vi "white line 2.vi"   [LabVIEW 2010, in "Line Follower.lvrbt"]
uses:
  Line Follower.lvrbt
  <vilib>/NXT/Subs/MotorOutput.ctl
  <vilib>/NXT/Block Support/NXT_InputPort.ctl
  <vilib>/NXT/Dual Mode Library/Sensors/Light_On.vi
  <vilib>/NXT/Dual Mode Library/Display/drawNumber.vi
  <vilib>/NXT/Dual Mode Library/Waits/Wait_Num(msec).vi
  <vilib>/NXT/Dual Mode Library/Motors/MotorOn.vi
  <vilib>/NXT/Dual Mode Library/Motors/MotorBrake.vi
  <vilib>/NXT/Dual Mode Library/Sound/Tone.vi
  <vilib>/NXT/Dual Mode Library/Sensors/Sonar_cm.vi
types:
  T1 = typedef "LVHSConnector.ctl" = cluster{"Hardware":string, "Flattened String":string}
  T2 = typedef "MotorOutput.ctl" = u8
  T3 = typedef "NXT_InputPort.ctl" = u8
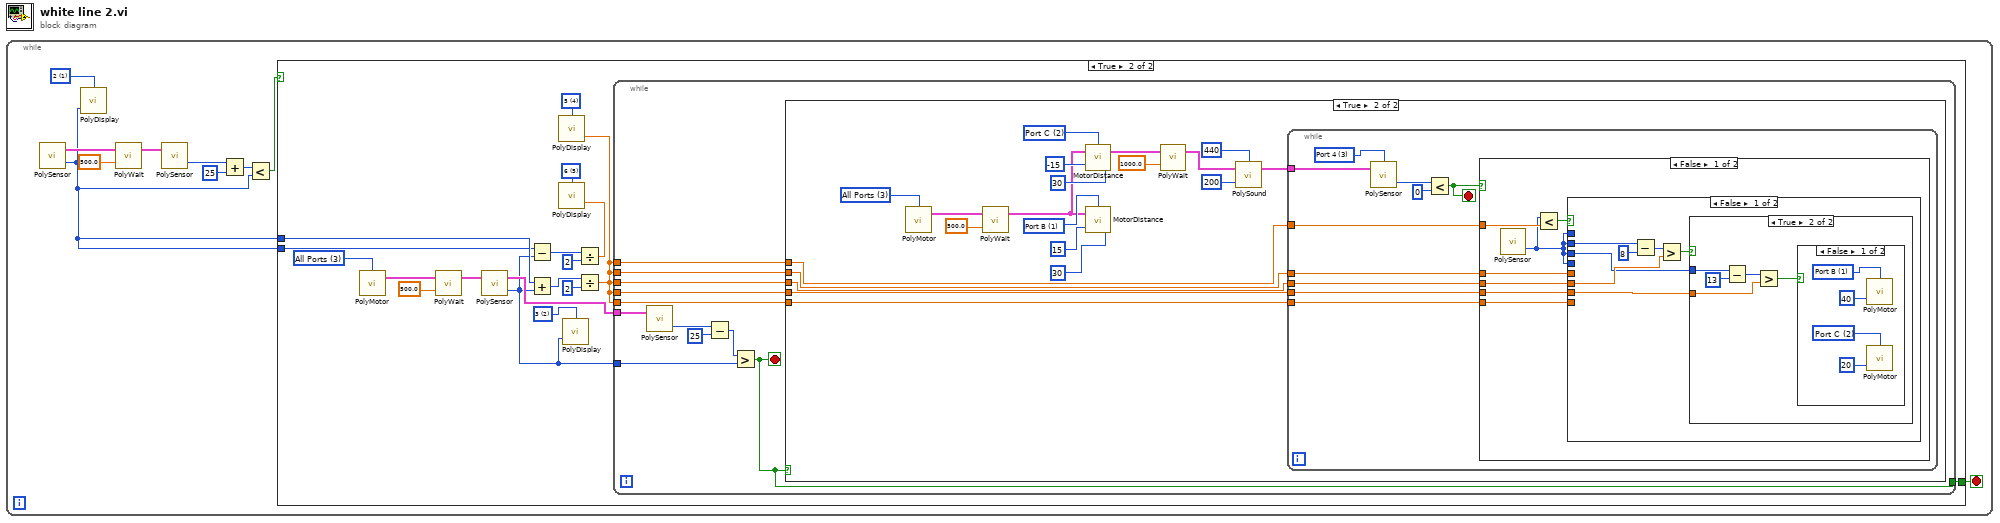
[diagram p0: block diagram]
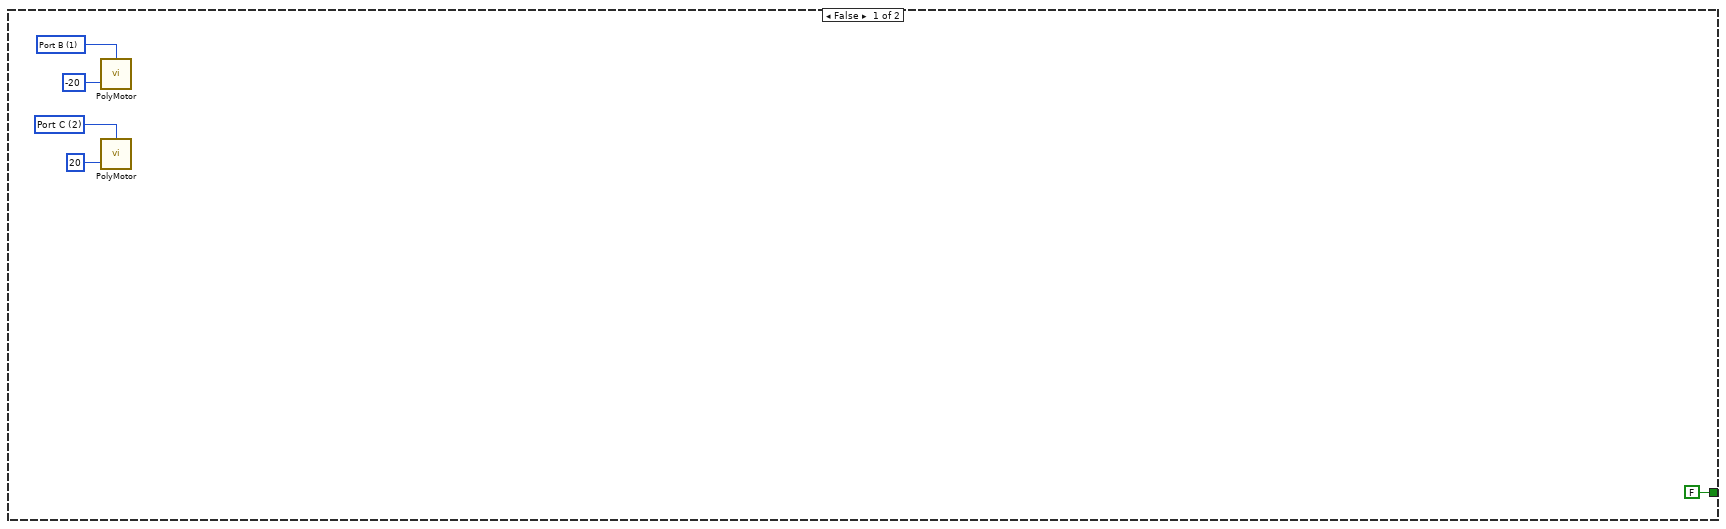
[diagram p2: hidden frame]
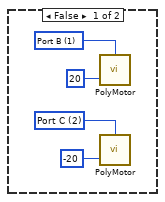
[diagram p3: hidden frame]
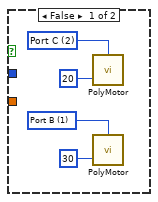
[diagram p4: hidden frame]
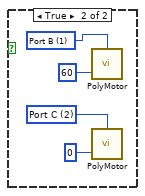
[diagram p5: hidden frame]
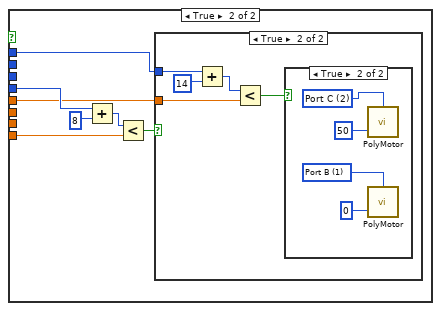
[diagram p6: hidden frame]
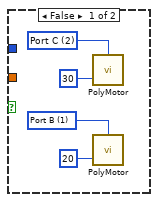
[diagram p7: hidden frame]
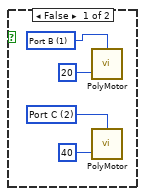
[diagram p8: hidden frame]
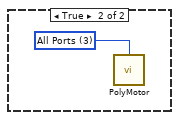
[diagram p9: hidden frame]
diagram:
  n1 = while {
    stop <- w2 stop-if-true
    w4 = i16 1 items=["1", "2", "3", "4", "5", "6", "7", "8"] ("Line")
    n2 = call-poly <vilib>:"PolySensor.vi"() -> ("Scaled Value"=w1:i16, "NXT"=w7:T1)  [unwired: 3 in]
    n3 = call-poly <vilib>:"PolyDisplay.vi"("number"=w1, "Line"=w4) -> ()  [unwired: 2 in, 1 out]
    n4 = call-poly <vilib>:"PolyWait.vi"("Time (100 msec)"=sgl 500.0 ("Time (1 sec)"), "NXT"=w7) -> ("NXT"=w6:T1)  [unwired: 2 in]
    n5 = call-poly <vilib>:"PolySensor.vi"("NXT"=w6) -> ("Scaled Value"=w9:i16)  [unwired: 2 in, 1 out]
    n6 = Add(x=w9, y=i16 25) -> (x+y=w3:i16)
    n7 = Less?(x=w3, y=w1) -> (x < y?=w8:bool)
    n8 = case shown="True" w8 {
      tunnel: w1 -> [_ w28]
      tunnel: [FALSE w26] -> w2
      tunnel: w1 -> [_ w20]
      frame False {
        w13 = T2 1 items=["Port A"=0, "Port B"=1, "Port C"=2, "Ports A & B"=4, "Ports A & C"=5, "Ports B & C"=6, "All Ports"=3] ("Port (All Ports)")
        w15 = T2 2 items=["Port A"=0, "Port B"=1, "Port C"=2, "Ports A & B"=4, "Ports A & C"=5, "Ports B & C"=6, "All Ports"=3] ("Output Port (All Ports)")
        n9 = call-poly <vilib>:"PolyMotor.vi"("Power (75)"=-20, "Output Port (All Ports)"=w13) -> ()  [unwired: 2 in, 1 out]
        n10 = call-poly <vilib>:"PolyMotor.vi"("Power (75)"=20, "Output Port (All Ports)"=w15) -> ()  [unwired: 2 in, 1 out]
      }
      frame True {
        w17 = i16 5 items=["1", "2", "3", "4", "5", "6", "7", "8"] ("Line")
        w29 = i16 2 items=["1", "2", "3", "4", "5", "6", "7", "8"] ("Line")
        w30 = i16 4 items=["1", "2", "3", "4", "5", "6", "7", "8"] ("Line")
        w33 = T2 3 items=["Port A"=0, "Port B"=1, "Port C"=2, "Ports A & B"=4, "Ports A & C"=5, "Ports B & C"=6, "All Ports"=3] ("Port (All Ports)")
        n11 = call-poly <vilib>:"PolyMotor.vi"("Port (All Ports)"=w33) -> ("NXT"=w24:T1)  [unwired: 3 in]
        n12 = call-poly <vilib>:"PolyWait.vi"("Time (100 msec)"=sgl 500.0 ("Time (1 sec)"), "NXT"=w24) -> ("NXT"=w23:T1)  [unwired: 2 in]
        n13 = call-poly <vilib>:"PolySensor.vi"("NXT"=w23) -> ("Scaled Value"=w19:i16, "NXT"=w22:T1)  [unwired: 2 in]
        n14 = Subtract(x=w20, y=w19) -> (x-y=w18:i16)
        n15 = Add(x=w28, y=w19) -> (x+y=w31:i16)
        n16 = call-poly <vilib>:"PolyDisplay.vi"("number"=w19, "Line"=w29) -> ()  [unwired: 2 in, 1 out]
        n17 = Divide(x=w18, y=i16 2) -> (x/y=w16:dbl)
        n18 = call-poly <vilib>:"PolyDisplay.vi"("number"=w16, "Line"=w17) -> ()  [unwired: 2 in, 1 out]
        n19 = Divide(x=w31, y=i16 2) -> (x/y=w25:dbl)
        n20 = call-poly <vilib>:"PolyDisplay.vi"("number"=w25, "Line"=w30) -> ()  [unwired: 2 in, 1 out]
        n21 = while {
          tunnel: w19 -> [w42]
          tunnel: w25 -> [w40]
          tunnel: w25 -> [w39]
          tunnel: w25 -> [w36]
          tunnel: w22 -> [w38]
          tunnel: [w37] -> w26
          tunnel: w25 -> [w35]
          tunnel: w25 -> [w34]
          stop <- w37 stop-if-true
          n22 = call-poly <vilib>:"PolySensor.vi"("NXT"=w38) -> ("Scaled Value"=w43:i16)  [unwired: 2 in, 1 out]
          n23 = Subtract(x=w43, y=i16 25) -> (x-y=w41:i16)
          n24 = Greater?(x=w41, y=w42) -> (0:w37:bool)
          n25 = case shown="True" w37 {
            tunnel: w40 -> [_ w58]
            tunnel: w39 -> [_ w57]
            tunnel: w36 -> [_ w56]
            tunnel: w35 -> [_ w53]
            tunnel: w34 -> [_ w52]
            frame False {
              w46 = T2 2 items=["Port A"=0, "Port B"=1, "Port C"=2, "Ports A & B"=4, "Ports A & C"=5, "Ports B & C"=6, "All Ports"=3] ("Port (All Ports)")
              w48 = T2 1 items=["Port A"=0, "Port B"=1, "Port C"=2, "Ports A & B"=4, "Ports A & C"=5, "Ports B & C"=6, "All Ports"=3] ("Output Port (All Ports)")
              n26 = call-poly <vilib>:"PolyMotor.vi"("Power (75)"=20, "Output Port (All Ports)"=w48) -> ()  [unwired: 2 in, 1 out]
              n27 = call-poly <vilib>:"PolyMotor.vi"("Power (75)"=-20, "Output Port (All Ports)"=w46) -> ()  [unwired: 2 in, 1 out]
            }
            frame True {
              w66 = T2 2 items=["Port A"=0, "Port B"=1, "Port C"=2, "Ports A & B"=4, "Ports A & C"=5, "Ports B & C"=6, "All Ports"=3] ("Port (All Ports)")
              w64 = T2 1 items=["Port A"=0, "Port B"=1, "Port C"=2, "Ports A & B"=4, "Ports A & C"=5, "Ports B & C"=6, "All Ports"=3] ("Output Port (All Ports)")
              w69 = T2 3 items=["Port A"=0, "Port B"=1, "Port C"=2, "Ports A & B"=4, "Ports A & C"=5, "Ports B & C"=6, "All Ports"=3] ("Port (All Ports)")
              n28 = call-poly <vilib>:"PolyMotor.vi"("Port (All Ports)"=w69) -> ("NXT"=w59:T1)  [unwired: 3 in]
              n29 = call-poly <vilib>:"PolyWait.vi"("Time (100 msec)"=sgl 500.0 ("Time (1 sec)"), "NXT"=w59) -> ("NXT"=w61:T1)  [unwired: 2 in]
              n30 = call <vilib>:"MotorDistance.vi"("Power (75)"=-15, "Angle of Rotation (360)"=30, "NXT"=w61, "Output Port (All Ports)"=w66) -> ("NXT"=w51:T1)
              n31 = call <vilib>:"MotorDistance.vi"("Power (75)"=15, "Angle of Rotation (360)"=30, "NXT"=w61, "Output Port (All Ports)"=w64) -> ()  [unwired: 1 out]
              n32 = call-poly <vilib>:"PolyWait.vi"("Time (100 msec)"=sgl 1000.0 ("Time (1 sec)"), "NXT"=w51) -> ("NXT"=w50:T1)  [unwired: 2 in]
              n33 = call-poly <vilib>:"PolySound.vi"("Duration (500 ms)"=u16 200, "NXT"=w50, "Tone (440 Hz)"=u16 440) -> ("NXT"=w49:T1)  [unwired: 1 in]
              n34 = while {
                tunnel: w49 -> [w75]
                tunnel: w58 -> [w74]
                tunnel: w57 -> [w73]
                tunnel: w56 -> [w72]
                tunnel: w53 -> [w71]
                tunnel: w52 -> [w70]
                stop <- w77 stop-if-true
                w79 = T3 3 items=["Port 1", "Port 2", "Port 3", "Port 4"] ("Port (Port 4)")
                n35 = call-poly <vilib>:"PolySensor.vi"("NXT"=w75, "Port (Port 4)"=w79) -> ("Distance (cm)"=w78:i16)  [unwired: 1 in, 1 out]
                n36 = Less?(x=w78, y=i16 0) -> (x < y?=w77:bool)
                n37 = case shown="False" w77 {
                  tunnel: w74 -> [w85 _]
                  tunnel: w73 -> [w84 _]
                  tunnel: w72 -> [w83 _]
                  tunnel: w71 -> [w82 _]
                  tunnel: w70 -> [w80 _]
                  frame False {
                    n38 = call-poly <vilib>:"PolySensor.vi"() -> ("Scaled Value"=w81:i16)  [unwired: 3 in, 1 out]
                    n39 = Less?(x=w81, y=w85) -> (x < y?=w86:bool)
                    n40 = case shown="False" w86 {
                      tunnel: w81 -> [w90 _]
                      tunnel: w81 -> [_ w114]
                      tunnel: w84 -> [w89 _]
                      tunnel: w83 -> [_ w113]
                      tunnel: w81 -> [w88 _]
                      tunnel: w82 -> [w87 _]
                      tunnel: w81 -> [_ w112]
                      tunnel: w80 -> [_ w111]
                      frame False {
                        n41 = Subtract(x=w90, y=i16 8) -> (x-y=w91:i16)
                        n42 = Greater?(x=w91, y=w89) -> (0:w93:bool)
                        n43 = case shown="True" w93 {
                          tunnel: w88 -> [_ w102]
                          tunnel: w87 -> [_ w99]
                          frame False {
                            w96 = T2 2 items=["Port A"=0, "Port B"=1, "Port C"=2, "Ports A & B"=4, "Ports A & C"=5, "Ports B & C"=6, "All Ports"=3] ("Port (All Ports)")
                            w94 = T2 1 items=["Port A"=0, "Port B"=1, "Port C"=2, "Ports A & B"=4, "Ports A & C"=5, "Ports B & C"=6, "All Ports"=3] ("Output Port (All Ports)")
                            n44 = call-poly <vilib>:"PolyMotor.vi"("Power (75)"=20, "Output Port (All Ports)"=w96) -> ()  [unwired: 2 in, 1 out]
                            n45 = call-poly <vilib>:"PolyMotor.vi"("Power (75)"=30, "Output Port (All Ports)"=w94) -> ()  [unwired: 2 in, 1 out]
                          }
                          frame True {
                            n46 = Subtract(x=w102, y=i16 13) -> (x-y=w100:i16)
                            n47 = Greater?(x=w100, y=w99) -> (0:w98:bool)
                            n48 = case shown="False" w98 {
                              frame False {
                                w105 = T2 2 items=["Port A"=0, "Port B"=1, "Port C"=2, "Ports A & B"=4, "Ports A & C"=5, "Ports B & C"=6, "All Ports"=3] ("Port (All Ports)")
                                w103 = T2 1 items=["Port A"=0, "Port B"=1, "Port C"=2, "Ports A & B"=4, "Ports A & C"=5, "Ports B & C"=6, "All Ports"=3] ("Output Port (All Ports)")
                                n49 = call-poly <vilib>:"PolyMotor.vi"("Power (75)"=40, "Output Port (All Ports)"=w103) -> ()  [unwired: 2 in, 1 out]
                                n50 = call-poly <vilib>:"PolyMotor.vi"("Power (75)"=20, "Output Port (All Ports)"=w105) -> ()  [unwired: 2 in, 1 out]
                              }
                              frame True {
                                w109 = T2 2 items=["Port A"=0, "Port B"=1, "Port C"=2, "Ports A & B"=4, "Ports A & C"=5, "Ports B & C"=6, "All Ports"=3] ("Port (All Ports)")
                                w107 = T2 1 items=["Port A"=0, "Port B"=1, "Port C"=2, "Ports A & B"=4, "Ports A & C"=5, "Ports B & C"=6, "All Ports"=3] ("Output Port (All Ports)")
                                n51 = call-poly <vilib>:"PolyMotor.vi"("Power (75)"=60, "Output Port (All Ports)"=w107) -> ()  [unwired: 2 in, 1 out]
                                n52 = call-poly <vilib>:"PolyMotor.vi"("Power (75)"=0, "Output Port (All Ports)"=w109) -> ()  [unwired: 2 in, 1 out]
                              }
                            }
                          }
                        }
                      }
                      frame True {
                        n53 = Add(x=w114, y=i16 8) -> (x+y=w116:i16)
                        n54 = Less?(x=w116, y=w113) -> (x < y?=w115:bool)
                        n55 = case shown="True" w115 {
                          tunnel: w112 -> [_ w126]
                          tunnel: w111 -> [_ w124]
                          frame False {
                            w121 = T2 1 items=["Port A"=0, "Port B"=1, "Port C"=2, "Ports A & B"=4, "Ports A & C"=5, "Ports B & C"=6, "All Ports"=3] ("Port (All Ports)")
                            w119 = T2 2 items=["Port A"=0, "Port B"=1, "Port C"=2, "Ports A & B"=4, "Ports A & C"=5, "Ports B & C"=6, "All Ports"=3] ("Output Port (All Ports)")
                            n56 = call-poly <vilib>:"PolyMotor.vi"("Power (75)"=30, "Output Port (All Ports)"=w119) -> ()  [unwired: 2 in, 1 out]
                            n57 = call-poly <vilib>:"PolyMotor.vi"("Power (75)"=20, "Output Port (All Ports)"=w121) -> ()  [unwired: 2 in, 1 out]
                          }
                          frame True {
                            n58 = Add(x=w126, y=i16 14) -> (x+y=w123:i16)
                            n59 = Less?(x=w123, y=w124) -> (x < y?=w122:bool)
                            n60 = case shown="True" w122 {
                              frame False {
                                w129 = T2 1 items=["Port A"=0, "Port B"=1, "Port C"=2, "Ports A & B"=4, "Ports A & C"=5, "Ports B & C"=6, "All Ports"=3] ("Port (All Ports)")
                                w127 = T2 2 items=["Port A"=0, "Port B"=1, "Port C"=2, "Ports A & B"=4, "Ports A & C"=5, "Ports B & C"=6, "All Ports"=3] ("Output Port (All Ports)")
                                n61 = call-poly <vilib>:"PolyMotor.vi"("Power (75)"=20, "Output Port (All Ports)"=w129) -> ()  [unwired: 2 in, 1 out]
                                n62 = call-poly <vilib>:"PolyMotor.vi"("Power (75)"=40, "Output Port (All Ports)"=w127) -> ()  [unwired: 2 in, 1 out]
                              }
                              frame True {
                                w133 = T2 1 items=["Port A"=0, "Port B"=1, "Port C"=2, "Ports A & B"=4, "Ports A & C"=5, "Ports B & C"=6, "All Ports"=3] ("Port (All Ports)")
                                w131 = T2 2 items=["Port A"=0, "Port B"=1, "Port C"=2, "Ports A & B"=4, "Ports A & C"=5, "Ports B & C"=6, "All Ports"=3] ("Output Port (All Ports)")
                                n63 = call-poly <vilib>:"PolyMotor.vi"("Power (75)"=50, "Output Port (All Ports)"=w131) -> ()  [unwired: 2 in, 1 out]
                                n64 = call-poly <vilib>:"PolyMotor.vi"("Power (75)"=0, "Output Port (All Ports)"=w133) -> ()  [unwired: 2 in, 1 out]
                              }
                            }
                          }
                        }
                      }
                    }
                  }
                  frame True {
                    w135 = T2 3 items=["Port A"=0, "Port B"=1, "Port C"=2, "Ports A & B"=4, "Ports A & C"=5, "Ports B & C"=6, "All Ports"=3] ("Port (All Ports)")
                    n65 = call-poly <vilib>:"PolyMotor.vi"("Port (All Ports)"=w135) -> ()  [unwired: 3 in, 1 out]
                  }
                }
              }
            }
          }
        }
      }
    }
  }
